vi "Deg_Rad.vi"(1 "Angle":dbl format="%.2f") -> (0 "RadRot":dbl format="%.9f")   [LabVIEW 2019]
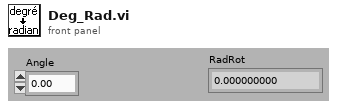
[diagram p1: front panel]
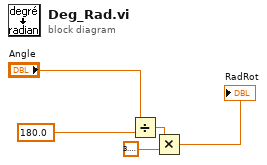
[diagram p0: block diagram]
diagram:
  n1 = Divide(x="Angle", y=180.0) -> (x/y=w4:dbl)
  n2 = Multiply(x=w4, y=3.141592653589793) -> (x*y=→"RadRot":dbl)
